vi "VISA to TCP.vi"(8 "Error In":errorcluster, 11 "VISA resource name":refnum<visa-resource-name>) -> (0 "Error Out":errorcluster, 1 "Port":u16, 2 "Hostname":string, 3 "VISA resource name out":refnum<visa-resource-name>)   [LabVIEW 2016]
panel:
  out "substring":string
  out "before substring":string
  out "General Settings:Resource Name":string
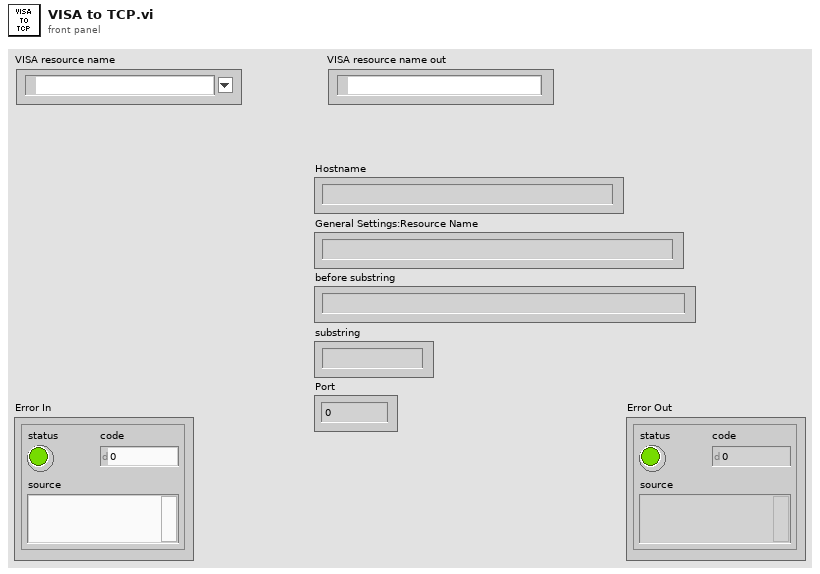
[diagram p1: front panel]
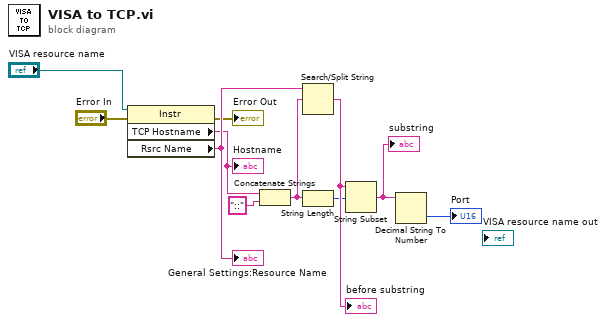
[diagram p0: block diagram]
diagram:
  n1 = property class="Instr"(reference="VISA resource name", error in="Error In") -> (error out=→"Error Out":errorcluster, "TCP Hostname"=w7:string, "Rsrc Name"=w8:string)  [unwired: 1 out]
  "Hostname" <- w7
  "General Settings:Resource Name" <- w8
  n2 = Concatenate Strings(w7, "::" ("string")) -> (w5:string)
  n3 = Search/Split String(string=w8, search string/char (-)=w5) -> (match + rest of string=w6:string)  [unwired: 1 in, 2 out]
  "before substring" <- w6
  n4 = String Length(string=w5) -> (length=w4:i32)
  n5 = String Subset(string=w6, offset (0)=w4) -> (substring=w3:string)  [unwired: 1 in]
  "substring" <- w3
  n6 = Decimal String To Number(string=w3) -> (number=→"Port":i32)  [unwired: 2 in, 1 out]
